vi "Multiply - CM,CM.vi"(1 "Complex Matrix B":T1, 2 "Complex Matrix A":T1) -> (0 "A * B":T1)   [LabVIEW 2018, in "NI_Matrix.lvlib"]
doc: "Returns the product of the inputs."
uses:
  NI_Matrix.lvlib
  ComplexMatrix.ctl
  Complex A x B.vi
  NI_AALBase.lvlib
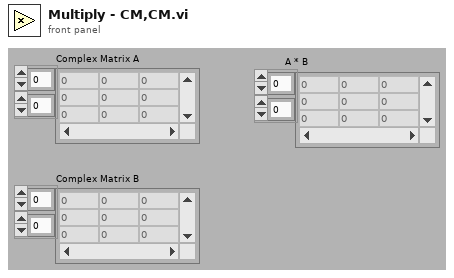
[diagram p1: front panel]
types:
  T1 = typedef "NI_Matrix.lvlib/ComplexMatrix.ctl" = cdb[][]
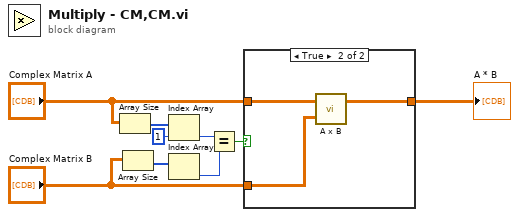
[diagram p0: block diagram]
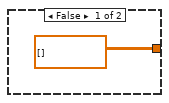
[diagram p2: hidden frame]
diagram:
  n1 = Array Size(array="Complex Matrix A") -> (size(s)=w5:i32[])
  n2 = Array Size(array="Complex Matrix B") -> (size(s)=w4:i32[])
  n3 = Index Array(array=w5, index=1) -> (element=w1:i32)
  n4 = Index Array(array=w4) -> (element=w2:i32)  [unwired: 1 in]
  n5 = Equal?(x=w1, y=w2) -> (x = y?=w9:bool)
  n6 = case shown="True" w9 {
    tunnel: "Complex Matrix A" -> [_ w13]
    tunnel: "Complex Matrix B" -> [_ w12]
    tunnel: [T1 [] ("A + B") w11] -> w6
    frame False {
    }
    frame True {
      n7 = call-poly "A x B.vi"("B"=w12, "A"=w13) -> ("A x B"=w11:T1)  [unwired: 1 out]
    }
  }
  "A * B" <- w6
